vi "RT_BLOGIC_Ramp.vi"(8 "Err_In":errorcluster, 10 "Data_In":T2={"Clck"=0, "Accel_Rt"=0.0, "Decel_Rt"=0.0, "Fin_Val"=0.0, "Hold"=TRUE, "Byp"=TRUE}) -> (0 "Err_Out":errorcluster, 2 "Data_Out":T1)   [LabVIEW 2024]
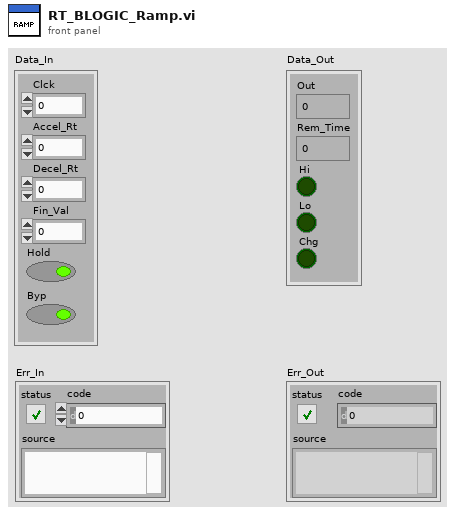
[diagram p1: front panel]
types:
  T1 = cluster{"Out":sgl, "Rem_Time":sgl, "Hi":bool, "Lo":bool, "Chg":bool}
  T2 = cluster{"Clck":u32, "Accel_Rt":sgl, "Decel_Rt":sgl, "Fin_Val":sgl, "Hold":bool, "Byp":bool}
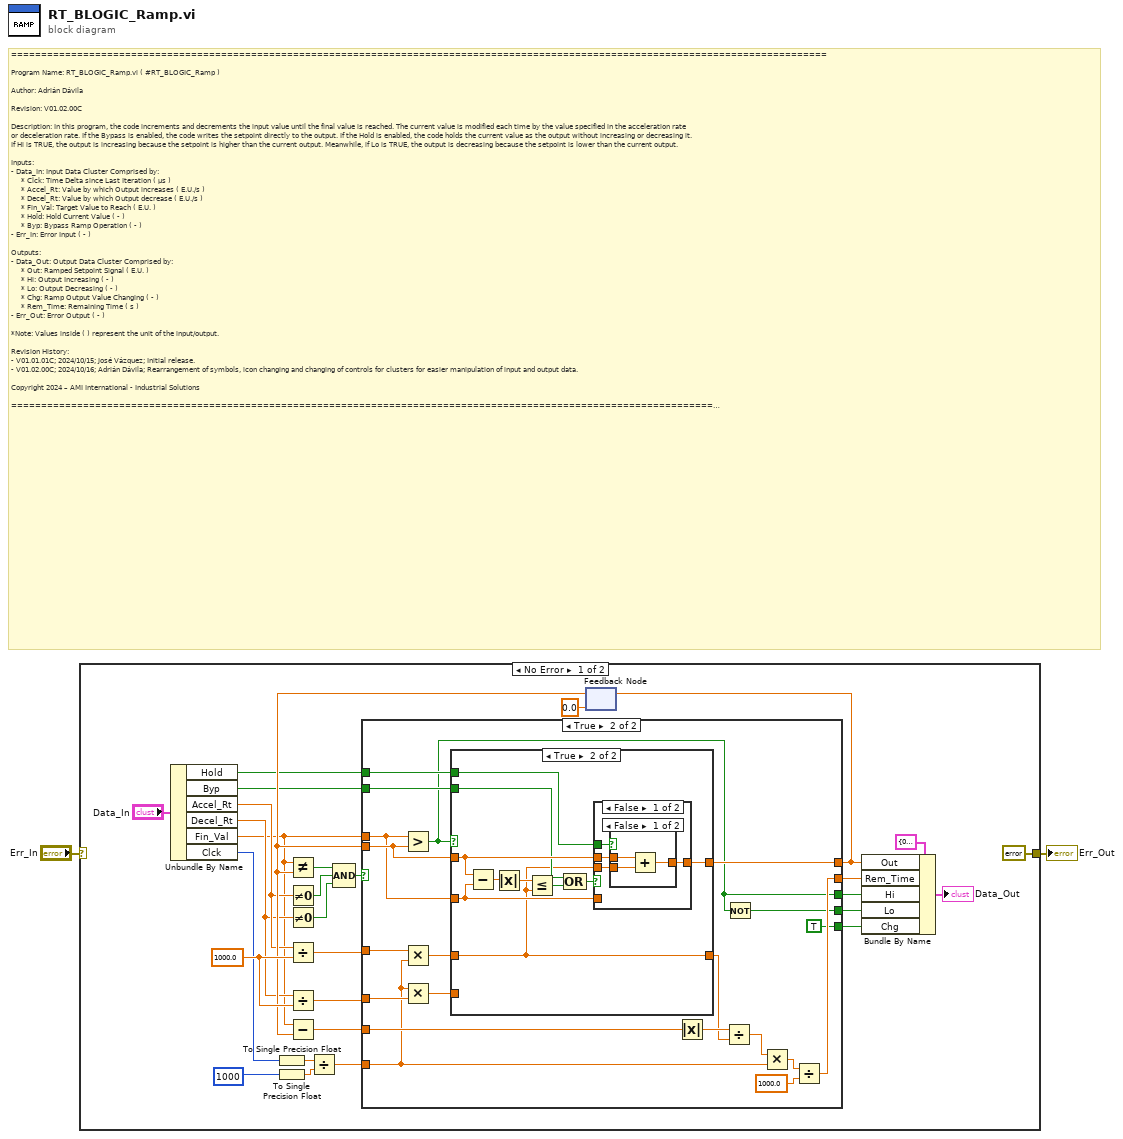
[diagram p0: block diagram]
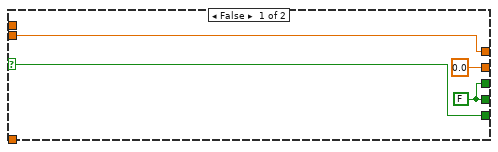
[diagram p2: hidden frame]
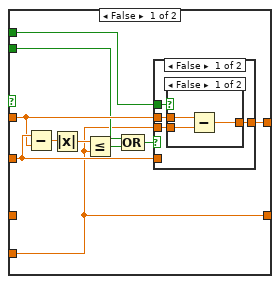
[diagram p3: hidden frame]
diagram:
  # "========================================================================================================================================\n\nProgram Name: RT_BLOGIC_Ramp.vi ( #RT_BLOGIC_Ramp )\n\nAuthor: Adrián Dávila\n\nRevision: V01.02.00C\n\nDescription: In this program, the code increments and decrements the input value until the final value is reached. The current value is modified each time by the value specified in the acceleration rate\nor deceleration rate. If the Bypass is enabled, the code writes the setpoint directly to the output. If the Hold is enabled, the code holds the current value as the output without increasing or decreasing it.\nIf Hi is TRUE, the output is increasing because the setpoint is higher than the current output. Meanwhile, if Lo is TRUE, the output is decreasing because the setpoint is lower than the current output.\n\nInputs:\n- Data_In: Input Data Cluster Comprised by:\n     * Clck: Time Delta since Last Iteration ( µs )\n     * Accel_Rt: Value by which Output increases ( E.U./s )\n     * Decel_Rt: Value by which Output decrease ( E.U./s )\n     * Fin_Val: Target Value to Reach ( E.U. )\n     * Hold: Hold Current Value ( - )\n     * Byp: Bypass Ramp Operation ( - )\n- Err_In: Error Input ( - )\n\nOutputs:\n- Data_Out: Output Data Cluster Comprised by:\n     * Out: Ramped Setpoint Signal ( E.U. )\n     * Hi: Output Increasing ( - )\n     * Lo: Output Decreasing ( - )\n     * Chg: Ramp Output Value Changing ( - )\n     * Rem_Time: Remaining Time ( s )\n- Err_Out: Error Output ( - )\n\n*Note: Values inside ( ) represent the unit of the input/output.\n \nRevision History: \n- V01.01.01C; 2024/10/15; José Vázquez; Initial release.\n- V01.02.00C; 2024/10/16; Adrián Dávila; Rearrangement of symbols, icon changing and changing of controls for clusters for easier manipulation of input and output data.\n\nCopyright 2024 – AMI International - Industrial Solutions\n\n========================================================================================================================================"
  n1 = case shown="No Error" "Err_In" {
    selector: "Err_In" -> [_ w94]
    tunnel: [errorcluster {"status"=FALSE, "code"=0, "source"=""} ("error IO") w94] -> w1
    frame No Error {
      w28 = sgl 1000.0
      n2 = Unbundle By Name("Data_In") -> ("Hold"=w13:bool, "Byp"=w12:bool, "Accel_Rt"=w17:sgl, "Decel_Rt"=w16:sgl, "Fin_Val"=w15:sgl, "Clck"=w14:u32)
      n3 = To Single Precision Float(number=w14) -> (single precision float=w25:sgl)
      n4 = To Single Precision Float(number=u32 1000 ("y")) -> (single precision float=w23:sgl)
      n5 = Not Equal To 0?(x=w17) -> (x != 0?=w31:bool)
      n6 = Not Equal To 0?(x=w16) -> (x != 0?=w30:bool)
      n7 = Divide(x=w17, y=w28) -> (x/y=w27:sgl)
      n8 = Divide(x=w16, y=w28) -> (x/y=w26:sgl)
      n9 = Divide(x=w25, y=w23) -> (x/y=w19:sgl)
      n10 = feedback #1(sgl 0.0 ("Setpoint")) -> (w21:sgl)
      n11 = Not Equal?(x=w15, y=w21) -> (x != y?=w29:bool)
      n12 = Subtract(x=w15, y=w21) -> (x-y=w22:sgl)
      n13 = Compound Arithmetic op=AND(w29, w31, w30) -> (w4:bool)
      n14 = case shown="True" w4 {
        selector: w4 -> [w32 _]
        tunnel: w27 -> [_ w51]
        tunnel: w26 -> [_ w50]
        tunnel: w15 -> [_ w49]
        tunnel: w21 -> [w35 w55]
        tunnel: [w35 w54] -> w9
        tunnel: w12 -> [_ w48]
        tunnel: w22 -> [_ w46]
        tunnel: w13 -> [_ w42]
        tunnel: w19 -> [_ w41]
        tunnel: [sgl 0.0 w40] -> w8
        tunnel: [w33 w36] -> w7
        tunnel: [w33 w39] -> w6
        tunnel: [w32 TRUE] -> w3
        frame False {
          w33 = FALSE ("Lower")
        }
        frame True {
          n15 = Greater?(x=w49, y=w55) -> (0:w36:bool)
          n16 = Multiply(x=w51, y=w41) -> (x*y=w52:sgl)
          n17 = Multiply(x=w41, y=w50) -> (x*y=w53:sgl)
          n18 = case shown="True" w36 {
            tunnel: w55 -> [w61 w80]
            tunnel: [w65 w84] -> w54
            tunnel: w53 -> [w56 _]
            tunnel: w52 -> [_ w75]
            tunnel: w49 -> [w62 w81]
            tunnel: w48 -> [w58 w77]
            tunnel: w42 -> [w57 w76]
            tunnel: [w56 w75] -> w38
            frame False {
              n19 = Subtract(x=w62, y=w61) -> (x-y=w64:sgl)
              n20 = Absolute Value(x=w64) -> (abs(x)=w63:sgl)
              n21 = Less Or Equal?(x=w63, y=w56) -> (x <= y?=w59:bool)
              n22 = Compound Arithmetic op=OR(w58, w59) -> (w60:bool)
              n23 = case shown="False" w60 {
                tunnel: [w69 w74] -> w65
                tunnel: w62 -> [_ w74]
                tunnel: w61 -> [w68 _]
                tunnel: w57 -> [w67 _]
                tunnel: w56 -> [w66 _]
                frame False {
                  n24 = case shown="False" w67 {
                    tunnel: w66 -> [w72 _]
                    tunnel: [w71 w73] -> w69
                    tunnel: w68 -> [w70 w73]
                    frame False {
                      n25 = Subtract(x=w70, y=w72) -> (x-y=w71:sgl)
                    }
                    frame True {
                    }
                  }
                }
                frame True {
                }
              }
            }
            frame True {
              n26 = Subtract(x=w80, y=w81) -> (x-y=w83:sgl)
              n27 = Absolute Value(x=w83) -> (abs(x)=w82:sgl)
              n28 = Less Or Equal?(x=w82, y=w75) -> (x <= y?=w79:bool)
              n29 = Compound Arithmetic op=OR(w77, w79) -> (w78:bool)
              n30 = case shown="False" w78 {
                tunnel: w81 -> [_ w93]
                tunnel: [w88 w93] -> w84
                tunnel: w80 -> [w87 _]
                tunnel: w76 -> [w86 _]
                tunnel: w75 -> [w85 _]
                frame False {
                  n31 = case shown="False" w86 {
                    tunnel: [w91 w92] -> w88
                    tunnel: w87 -> [w90 w92]
                    tunnel: w85 -> [w89 _]
                    frame False {
                      n32 = Add(x=w90, y=w89) -> (x+y=w91:sgl)
                    }
                    frame True {
                    }
                  }
                }
                frame True {
                }
              }
            }
          }
          n33 = Absolute Value(x=w46) -> (abs(x)=w47:sgl)
          n34 = Divide(x=w47, y=w38) -> (x/y=w45:sgl)
          n35 = Not(x=w36) -> (.not. x?=w39:bool)
          n36 = Multiply(x=w45, y=w41) -> (x*y=w44:sgl)
          n37 = Divide(x=w44, y=sgl 1000.0) -> (x/y=w40:sgl)
        }
      }
      n38 = feedback-in #1(w9) -> ()
      n39 = Bundle By Name(cluster=T1 {"Out"=0.0, "Rem_Time"=0.0, "Hi"=FALSE, "Lo"=FALSE, "Chg"=FALSE} ("Data_Out"), "Out"=w9, "Rem_Time"=w8, "Hi"=w7, "Lo"=w6, "Chg"=w3) -> (→"Data_Out":T1)
    }
    frame Error {
    }
  }
  "Err_Out" <- w1
